vi "Configure VNA.vi"(8 "error in (no error)":errorcluster, 10 "file path":path=path "C:/Users/Eddie.Rickey/Documents/RCV_PXI/Calibration/#Cal - VNA_ 50MHz.chx", 11 "Semiconductor Module Context":T1) -> (0 "error out":errorcluster)   [LabVIEW 2013]
uses:
  <vilib>/NI_TestStand_SemiconductorModule/NI_TestStand_Semiconductor_Module.lvlibp/PinMap/General/SemiconductorModuleContext.ctl
  <instrlib>/niVNA/niVNA.llb/niVNA Load Calibration And Configuration Data From File.vi
  Pin Map API/VNA Custom Instrument.lvlib
  <vilib>/NI_TestStand_SemiconductorModule/NI_TestStand_Semiconductor_Module.lvlibp
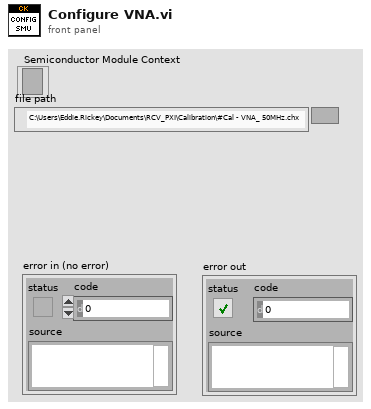
[diagram p1: front panel]
types:
  T1 = typedef "NI_TestStand_Semiconductor_Module.lvlibp/SemiconductorModuleContext.ctl" = refnum<k7>
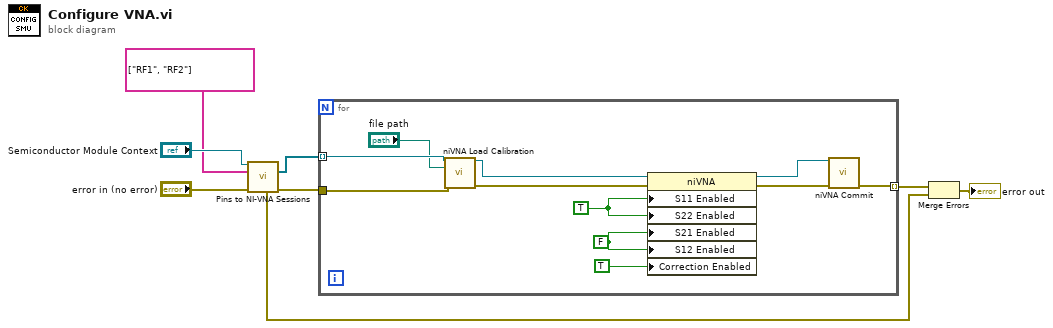
[diagram p0: block diagram]
diagram:
  n1 = call "Pins to NI-VNA Sessions.vi"("Semiconductor Module Context"="Semiconductor Module Context", "Pins"=string[] ["RF1", "RF2"], "error in (no error)"="error in (no error)") -> ("Instrument Sessions"=w2:refnum<k15>[], "error out"=w1:errorcluster)  [unwired: 8 in, 3 out]
  n2 = for {
    tunnel: w1 -> [w18]
    tunnel: [w8] -> w5 mode=indexing
    tunnel: w2 -> [w17] mode=indexing
    w12 = FALSE ("Sweep:S21 Enabled")
    w10 = TRUE ("Sweep:S11 Enabled")
    n3 = call-poly <instrlib>:"niVNA Load Calibration.vi"("instrument handle"=w17, "file path"="file path", "error in"=w18) -> ("instrument handle out"=w13:refnum<k15>, "error out"=w11:errorcluster)  [unwired: 11 in]
    n4 = property class="niVNA"(reference=w13, error in=w11, "S11 Enabled"=w10, "S22 Enabled"=w10, "S21 Enabled"=w12, "S12 Enabled"=w12, "Correction Enabled"=TRUE ("Calibration Settings:Correction Enabled")) -> (reference out=w14:refnum<k15>, error out=w15:errorcluster)
    n5 = call <instrlib>:"niVNA Commit.vi"("instrument handle"=w14, "error in"=w15) -> ("error out"=w8:errorcluster)  [unwired: 12 in, 1 out]
  }
  n6 = Merge Errors(w5, w1) -> (→"error out":errorcluster)
